vi "最高權限模式test.vi"() -> ()   [LabVIEW 2022 SP3]
panel:
  out "text":string[](array[string])
  out "Tab Control":enum32{"Page 1", "Page 2", "Page 3", "Page 4"}(tab)
  in  "輸入最高權限帳號:":string
  in  "輸入最高權限密碼:":string
  in  "登入":bool
  in  "Stop Button":bool
  in  "創建使用者帳號":bool
  in  "刪除使用者帳號":bool
  in  "登出":bool
  in  "創建密碼":string
  in  "創建帳號":string
  in  "創建建立":bool
  in  "創建離開":bool
  in  "Combo Box":string(combo)
  in  "刪除離開":bool
  in  "確認刪除":bool
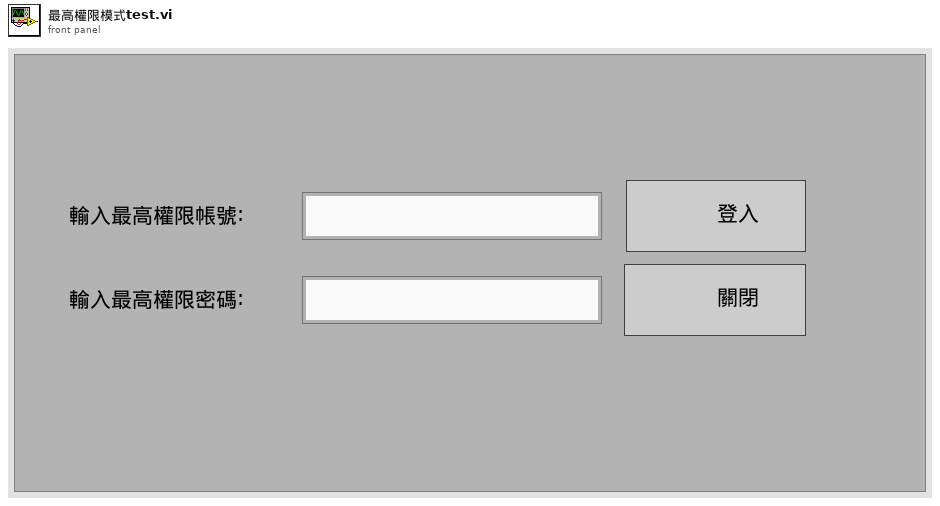
[diagram p1: front panel]
types:
  T1 = typedef "最高權限Control.ctl" = enum16{"刪除帳號", "創建帳號", "登出", "登入完成", "初始", "登入", "創建使用者帳密", "刪除使用者帳密", "離開"}
  T2 = enum16{"open", "replace", "create", "open or create", "replace or create", "replace or create with confirmation"}
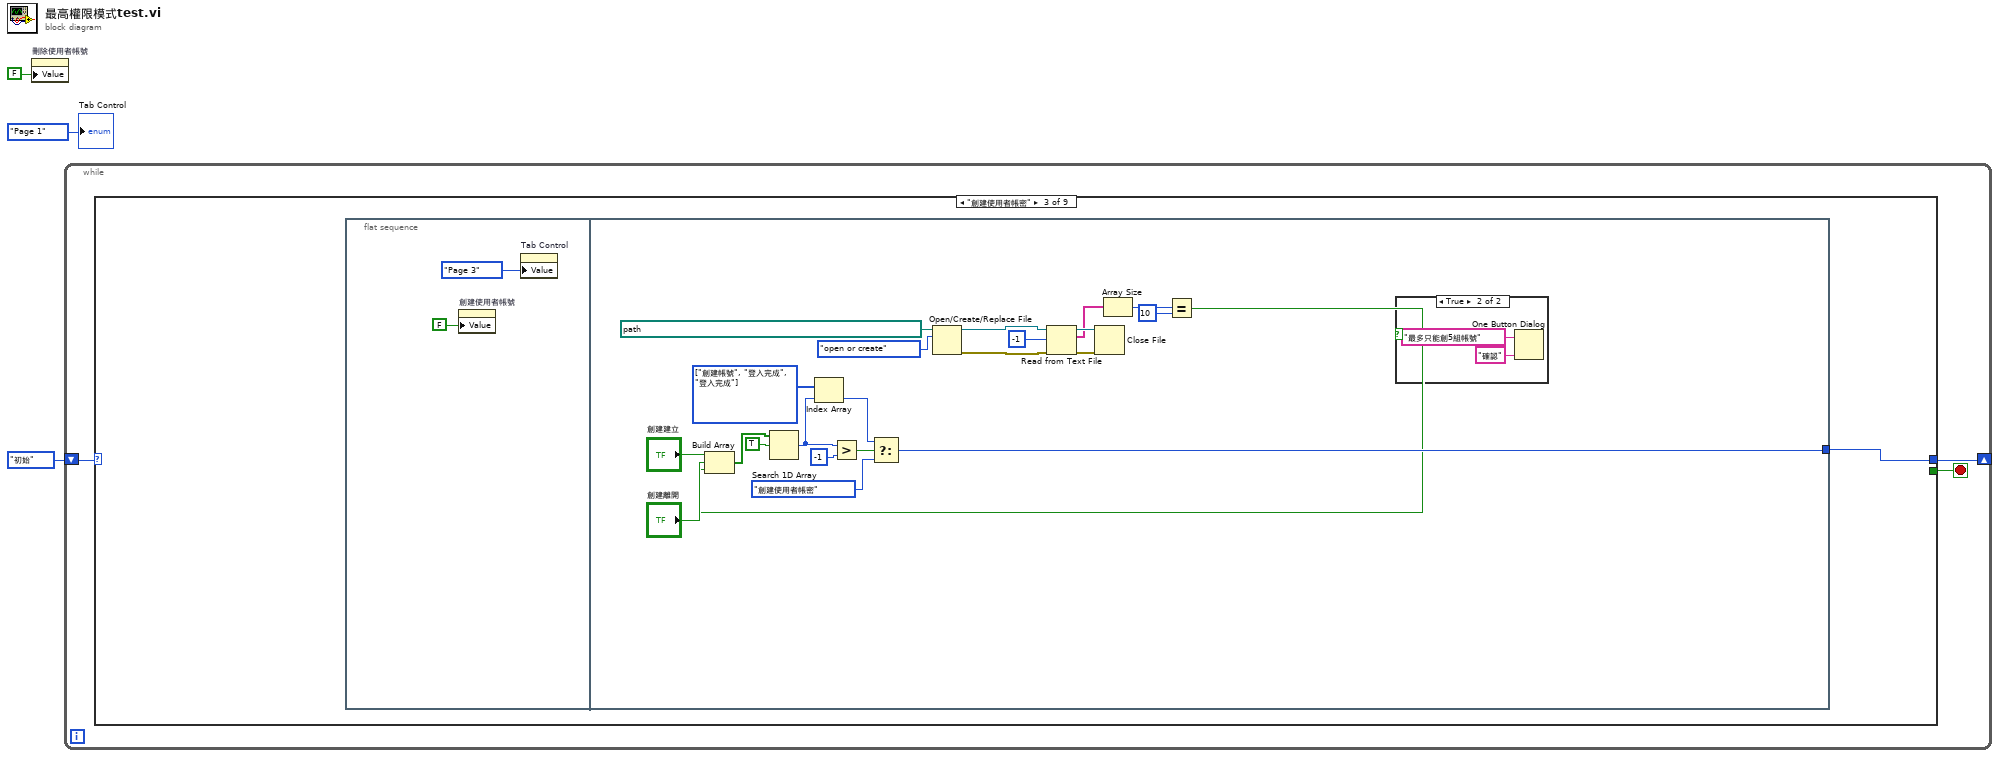
[diagram p0: block diagram]
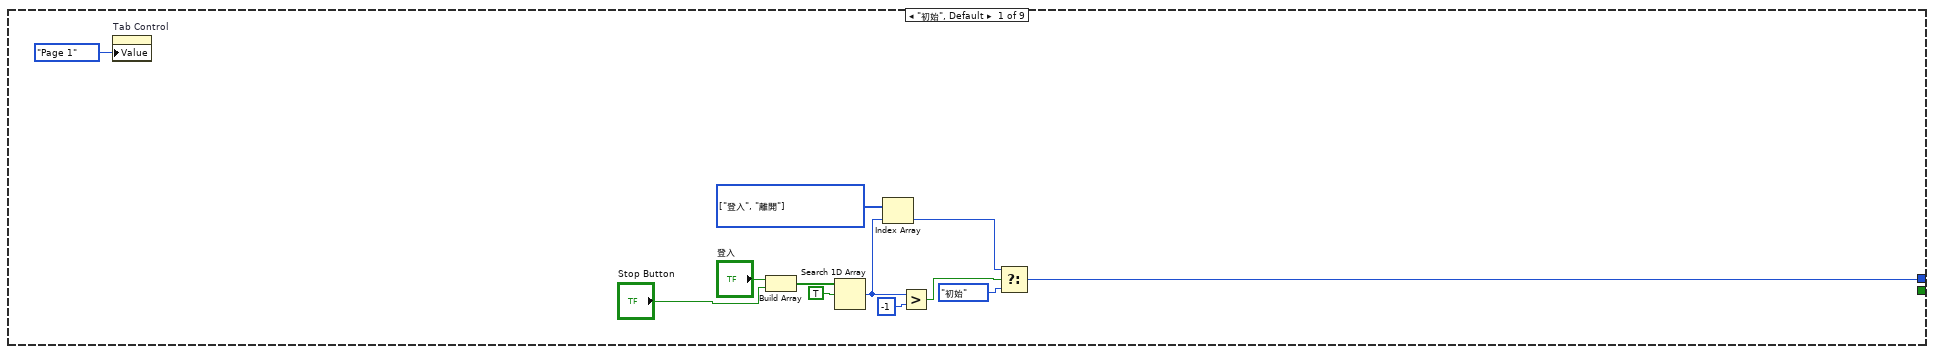
[diagram p2: hidden frame]
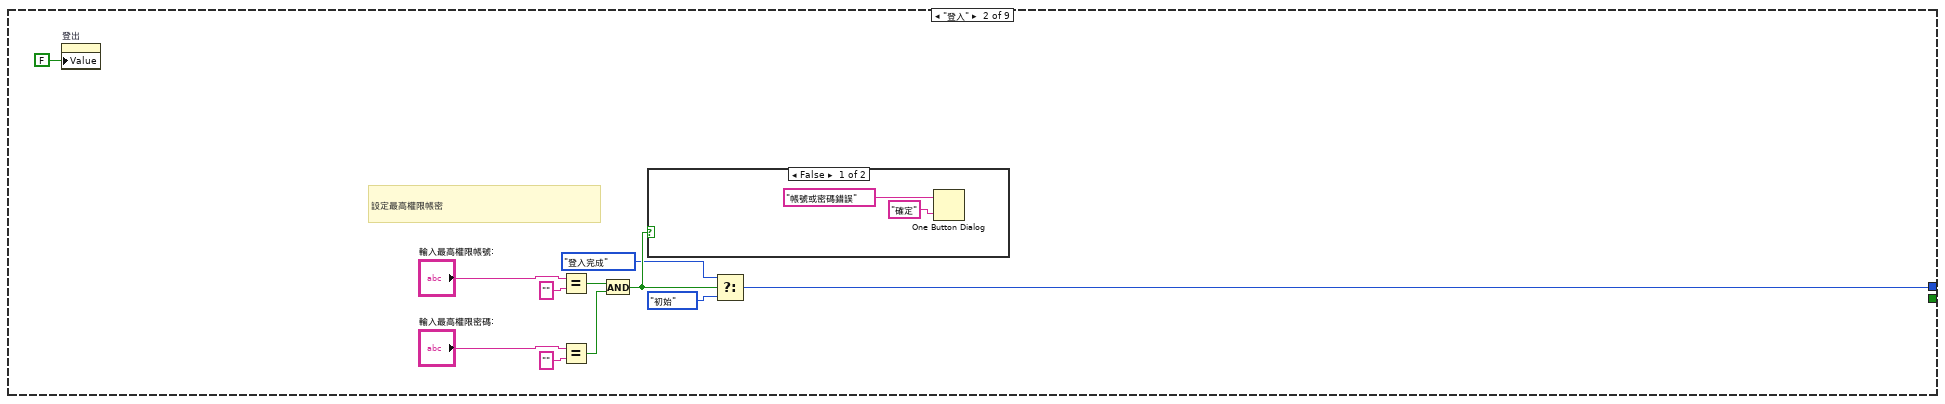
[diagram p3: hidden frame]
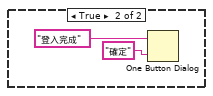
[diagram p4: hidden frame]
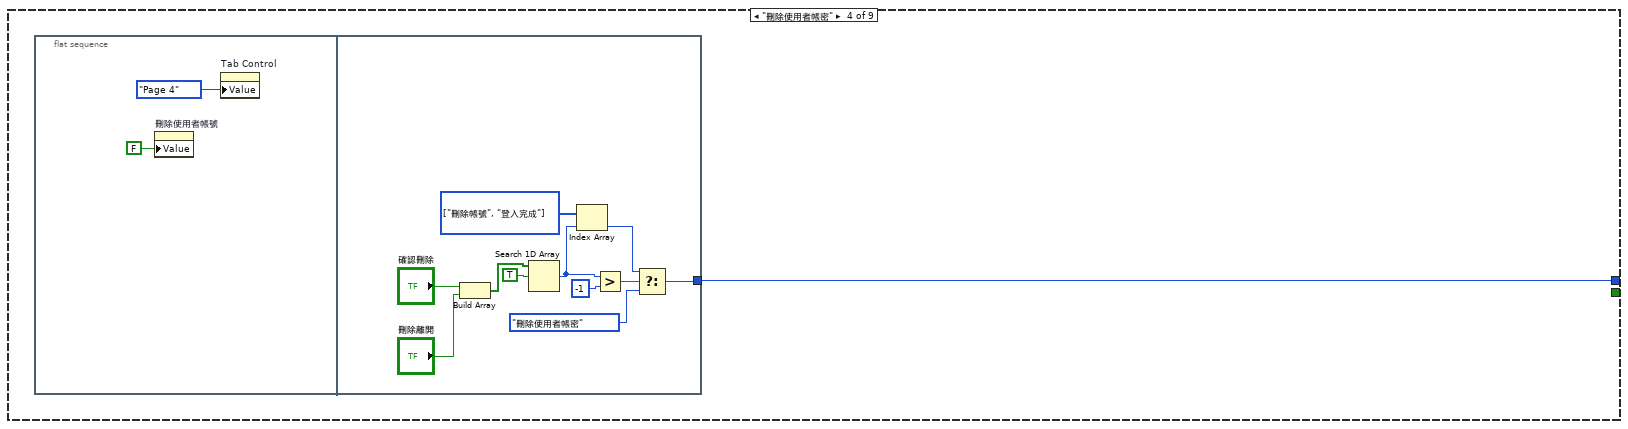
[diagram p6: hidden frame]
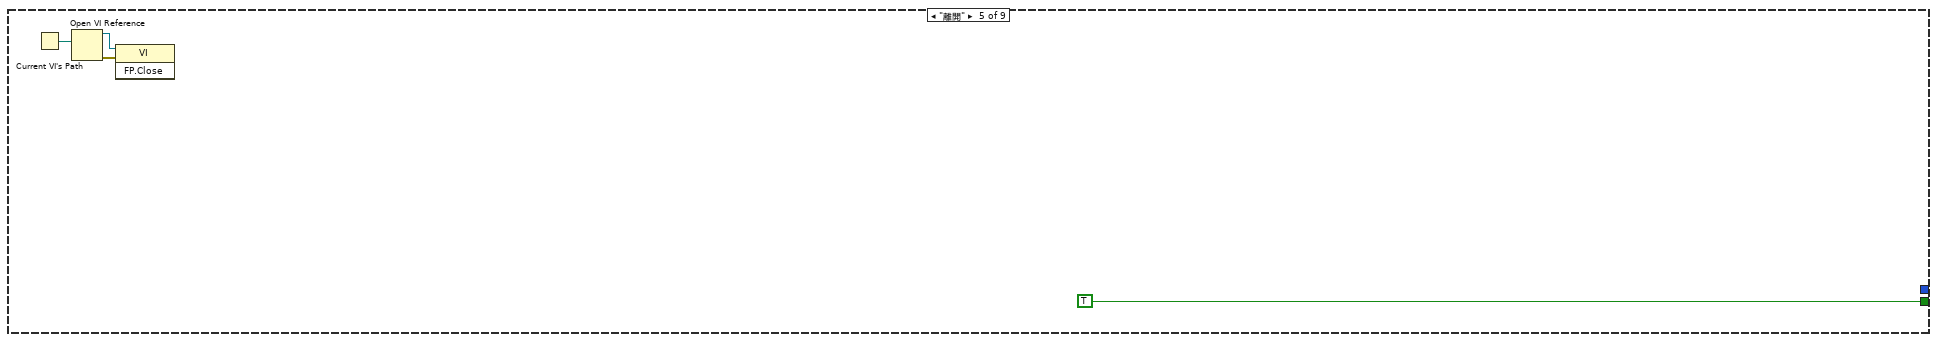
[diagram p7: hidden frame]
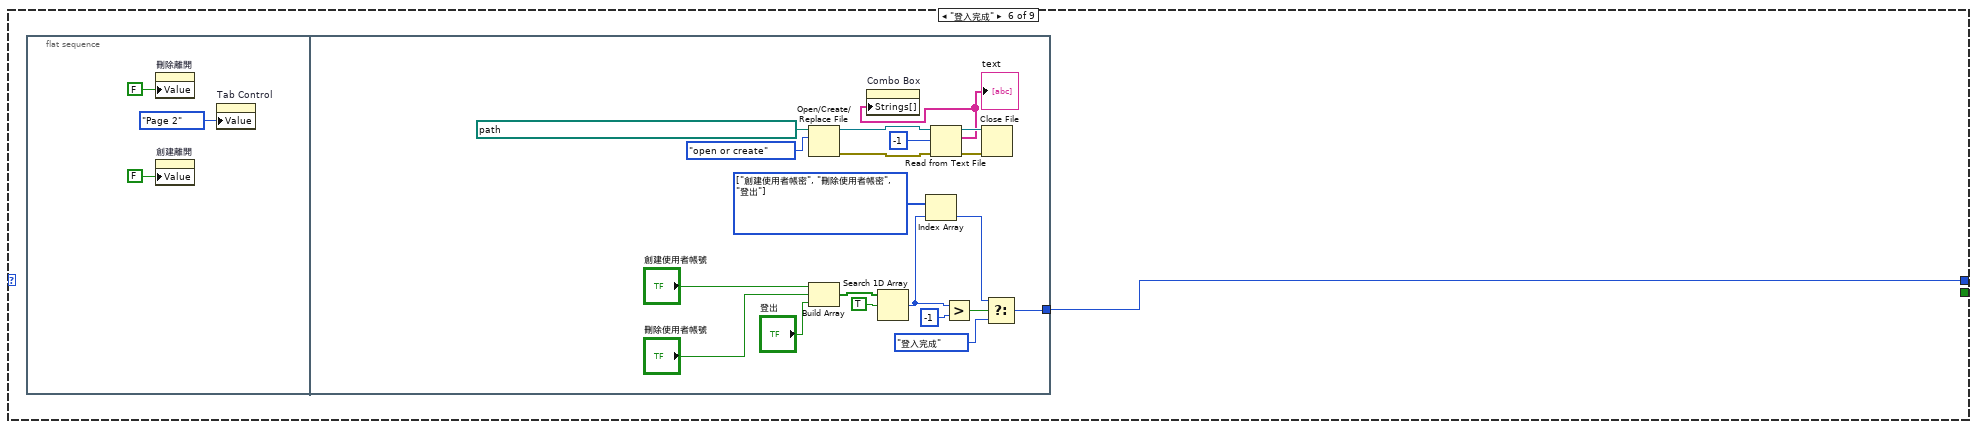
[diagram p8: hidden frame]
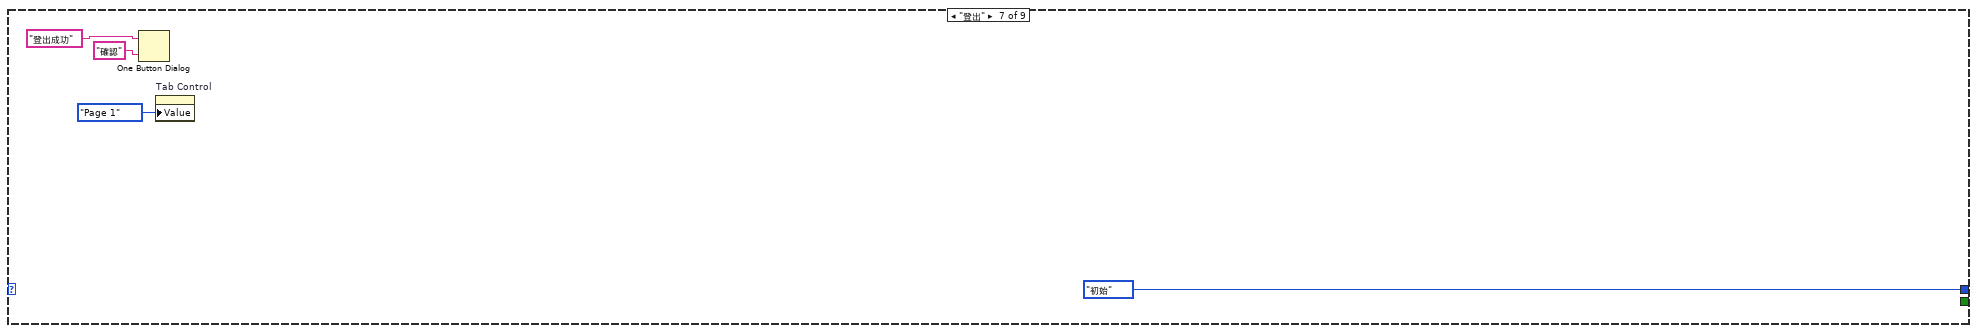
[diagram p9: hidden frame]
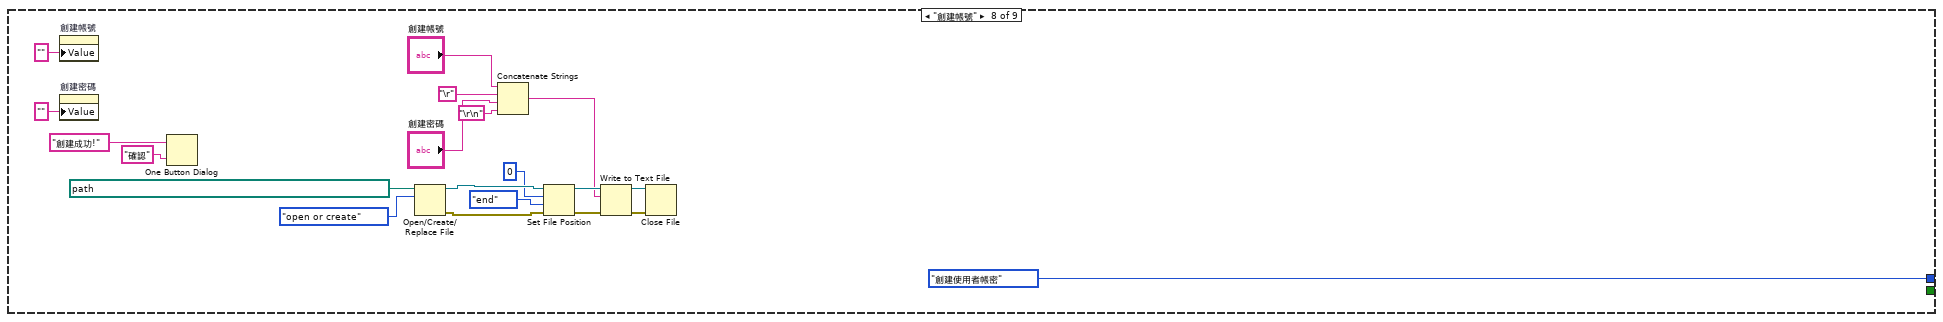
[diagram p10: hidden frame]
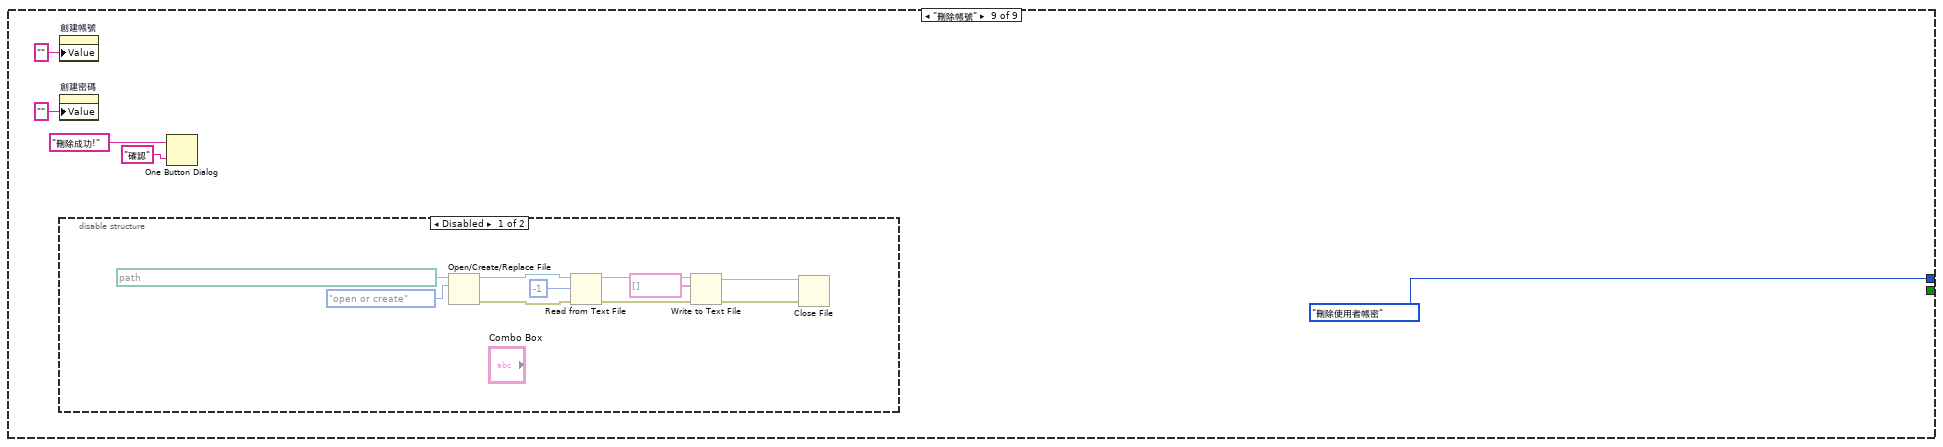
[diagram p11: hidden frame]
diagram:
  n1 = property on="刪除使用者帳號" class="Bool (strict)"("Value"=FALSE ("刪除使用者帳號")) -> ()  [unwired: 2 in, 2 out]
  n2 = while {
    shift-right: [w5] -> _
    shift-left: 最高權限Control."初始" -> [w6]
    stop <- w4 stop-if-true
    n3 = case shown="\"創建使用者帳密\"" w6 {
      tunnel: [w9 w20 w34 w61 _ w79 最高權限Control."初始" 最高權限Control."創建使用者帳密" 最高權限Control."刪除使用者帳密"] -> w5
      tunnel: [_ _ _ _ TRUE _ _ _ _] -> w4
      frame "初始", Default {
        w14 = T1[] [enum."登入", enum."離開"] items=["刪除帳號", "創建帳號", "登出", "登入完成", "初始", "登入", "創建使用者帳密", "刪除使用者帳密", "離開"]
        n4 = property on="Tab Control" class="TabCtl (strict)"("Value"=enum32{"Page 1", "Page 2"}."Page 1" ("Tab Control")) -> ()  [unwired: 2 in, 2 out]
        n5 = Build Array("登入", "Stop Button") -> (w16:bool[])
        n6 = Search 1D Array(1D array=w16, element=TRUE) -> (index of element=w13:i32)  [unwired: 1 in]
        n7 = Index Array(array=w14, index=w13) -> (element=w8:T1)
        n8 = Greater?(x=w13, y=-1) -> (0:w11:bool)
        n9 = Select(t=w8, s=w11, f=最高權限Control."初始") -> (s? t:f=w9:T1)
      }
      frame "登入" {
        # "設定最高權限帳密"
        n10 = property on="登出" class="Bool (strict)"("Value"=FALSE ("登出")) -> ()  [unwired: 2 in, 2 out]
        n11 = Equal?(x="輸入最高權限帳號:", y="") -> (x = y?=w25:bool)
        n12 = Equal?(x="輸入最高權限密碼:", y="") -> (x = y?=w24:bool)
        n13 = And(x=w25, y=w24) -> (x .and. y?=w23:bool)
        n14 = case shown="False" w23 {
          frame False {
            n15 = One Button Dialog(message="帳號或密碼錯誤", button name ("OK")="確定") -> ()  [unwired: 1 out]
          }
          frame True {
            n16 = One Button Dialog(message="登入完成", button name ("OK")="確定") -> ()  [unwired: 1 out]
          }
        }
        n17 = Select(t=最高權限Control."登入完成", s=w23, f=最高權限Control."初始") -> (s? t:f=w20:T1)
      }
      frame "創建使用者帳密" {
        n18 = flat-sequence {
          tunnel: [w48] -> w34
          frame #0 {
            n19 = property on="創建使用者帳號" class="Bool (strict)"("Value"=FALSE ("創建使用者帳號")) -> ()  [unwired: 2 in, 2 out]
            n20 = property on="Tab Control" class="TabCtl (strict)"("Value"=enum32{"Page 1", "Page 2", "Page 3", "Page 4"}."Page 3" ("Tab Control")) -> ()  [unwired: 2 in, 2 out]
          }
          frame #1 {
            w49 = T1[] [enum."創建帳號", enum."登入完成", enum."登入完成"] items=["刪除帳號", "創建帳號", "登出", "登入完成", "初始", "登入", "創建使用者帳密", "刪除使用者帳密", "離開"]
            n21 = Open/Create/Replace File(file path (use dialog)=path "C:/Users/kenny/OneDrive/桌面/機械手臂/使用者帳密.txt", operation (0:open)=T2."open or create") -> (refnum out=w44:refnum<file>, error out=w45:errorcluster)  [unwired: 4 in, 1 out]
            n22 = Read from Text File(file (use dialog)=w44, count=-1, error in=w45) -> (refnum out=w47:refnum<file>, text=w40:string[], error out=w46:errorcluster)  [unwired: 1 in, 1 out]
            n23 = Close File(refnum=w47, error in=w46) -> ()  [unwired: 2 out]
            n24 = Array Size(array=w40) -> (size(s)=w39:i32)
            n25 = Equal?(x=w39, y=10) -> (x = y?=w37:bool)
            n26 = Build Array("創建建立", "創建離開", w37) -> (w58:bool[])
            n27 = Search 1D Array(1D array=w58, element=TRUE) -> (index of element=w57:i32)  [unwired: 1 in]
            n28 = Index Array(array=w49, index=w57) -> (element=w55:T1)
            n29 = Greater?(x=w57, y=-1) -> (0:w56:bool)
            n30 = Select(t=w55, s=w56, f=最高權限Control."創建使用者帳密") -> (s? t:f=w48:T1)
            n31 = case shown="True" w37 {
              frame False {
              }
              frame True {
                n32 = One Button Dialog(message="最多只能創5組帳號", button name ("OK")="確認") -> ()  [unwired: 1 out]
              }
            }
          }
        }
      }
      frame "刪除使用者帳密" {
        n33 = flat-sequence {
          tunnel: [w64] -> w61
          frame #0 {
            n34 = property on="刪除使用者帳號" class="Bool (strict)"("Value"=FALSE ("刪除使用者帳號")) -> ()  [unwired: 2 in, 2 out]
            n35 = property on="Tab Control" class="TabCtl (strict)"("Value"=enum32{"Page 1", "Page 2", "Page 3", "Page 4"}."Page 4" ("Tab Control")) -> ()  [unwired: 2 in, 2 out]
          }
          frame #1 {
            w65 = T1[] [enum."刪除帳號", enum."登入完成"] items=["刪除帳號", "創建帳號", "登出", "登入完成", "初始", "登入", "創建使用者帳密", "刪除使用者帳密", "離開"]
            n36 = Build Array("確認刪除", "刪除離開") -> (w71:bool[])
            n37 = Search 1D Array(1D array=w71, element=TRUE) -> (index of element=w72:i32)  [unwired: 1 in]
            n38 = Index Array(array=w65, index=w72) -> (element=w74:T1)
            n39 = Greater?(x=w72, y=-1) -> (0:w73:bool)
            n40 = Select(t=w74, s=w73, f=最高權限Control."刪除使用者帳密") -> (s? t:f=w64:T1)
          }
        }
      }
      frame "離開" {
        n41 = Current VI's Path() -> (path=w75:path)
        n42 = Open VI Reference(vi path=w75) -> (vi reference=w77:refnum<vi>, error out=w76:errorcluster)  [unwired: 5 in]
        n43 = invoke class="VI" method="FP.Close"(reference=w77, error in=w76) -> ()  [unwired: 1 in, 3 out]
      }
      frame "登入完成" {
        n44 = flat-sequence {
          tunnel: [w91] -> w79
          frame #0 {
            n45 = property on="刪除離開" class="Bool (strict)"("Value"=FALSE ("刪除離開")) -> ()  [unwired: 2 in, 2 out]
            n46 = property on="創建離開" class="Bool (strict)"("Value"=FALSE ("創建離開")) -> ()  [unwired: 2 in, 2 out]
            n47 = property on="Tab Control" class="TabCtl (strict)"("Value"=enum32{"Page 1", "Page 2"}."Page 2" ("Tab Control")) -> ()  [unwired: 2 in, 2 out]
          }
          frame #1 {
            w92 = T1[] [enum."創建使用者帳密", enum."刪除使用者帳密", enum."登出"] items=["刪除帳號", "創建帳號", "登出", "登入完成", "初始", "登入", "創建使用者帳密", "刪除使用者帳密", "離開"]
            n48 = Open/Create/Replace File(file path (use dialog)=path "C:/Users/kenny/OneDrive/桌面/機械手臂/使用者帳密.txt", operation (0:open)=T2."open or create") -> (refnum out=w87:refnum<file>, error out=w88:errorcluster)  [unwired: 4 in, 1 out]
            n49 = Build Array("創建使用者帳號", "刪除使用者帳號", "登出") -> (w99:bool[])
            n50 = Search 1D Array(1D array=w99, element=TRUE) -> (index of element=w100:i32)  [unwired: 1 in]
            n51 = Index Array(array=w92, index=w100) -> (element=w101:T1)
            n52 = Read from Text File(file (use dialog)=w87, count=-1, error in=w88) -> (refnum out=w90:refnum<file>, text=w83:string[], error out=w89:errorcluster)  [unwired: 1 in, 1 out]
            "text" <- w83
            n53 = property on="Combo Box" class="CmbBox"("Strings[]"=w83) -> ()  [unwired: 2 in, 2 out]
            n54 = Greater?(x=w100, y=-1) -> (0:w102:bool)
            n55 = Close File(refnum=w90, error in=w89) -> ()  [unwired: 2 out]
            n56 = Select(t=w101, s=w102, f=最高權限Control."登入完成") -> (s? t:f=w91:T1)
          }
        }
      }
      frame "登出" {
        n57 = One Button Dialog(message="登出成功", button name ("OK")="確認") -> ()  [unwired: 1 out]
        n58 = property on="Tab Control" class="TabCtl (strict)"("Value"=enum32{"Page 1", "Page 2"}."Page 1" ("Tab Control")) -> ()  [unwired: 2 in, 2 out]
      }
      frame "創建帳號" {
        n59 = property on="創建帳號" class="Str"("Value"="" ("創建帳號")) -> ()  [unwired: 2 in, 2 out]
        n60 = property on="創建密碼" class="Str"("Value"="" ("創建密碼")) -> ()  [unwired: 2 in, 2 out]
        n61 = One Button Dialog(message="創建成功!", button name ("OK")="確認") -> ()  [unwired: 1 out]
        n62 = Open/Create/Replace File(file path (use dialog)=path "C:/Users/kenny/OneDrive/桌面/機械手臂/使用者帳密.txt", operation (0:open)=T2."open or create") -> (refnum out=w118:refnum<file>, error out=w116:errorcluster)  [unwired: 4 in, 1 out]
        n63 = Concatenate Strings("創建帳號", "\r", "創建密碼", "\r\n") -> (w109:string)
        n64 = Set File Position(offset (in bytes) (0)=i64 0, refnum=w118, from (0:start)=enum16{"start", "end", "current"}."end", error in=w116) -> (refnum out=w117:refnum<file>, error out=w115:errorcluster)
        n65 = Write to Text File(file (use dialog)=w117, text=w109, error in=w115) -> (refnum out=w122:refnum<file>, error out=w123:errorcluster)  [unwired: 1 in, 1 out]
        n66 = Close File(refnum=w122, error in=w123) -> ()  [unwired: 2 out]
      }
      frame "刪除帳號" {
        n67 = property on="創建帳號" class="Str"("Value"="" ("創建帳號")) -> ()  [unwired: 2 in, 2 out]
        n68 = property on="創建密碼" class="Str"("Value"="" ("創建密碼")) -> ()  [unwired: 2 in, 2 out]
        n69 = disable-structure shown="Disabled" {
          frame Disabled {
            n70 = Open/Create/Replace File(file path (use dialog)=path "C:/Users/kenny/OneDrive/桌面/機械手臂/使用者帳密.txt", operation (0:open)=T2."open or create") -> (refnum out=w140:refnum<file>, error out=w141:errorcluster)  [unwired: 4 in, 1 out]
            n71 = Read from Text File(file (use dialog)=w140, count=-1, error in=w141) -> (refnum out=w136:refnum<file>, error out=w135:errorcluster)  [unwired: 1 in, 2 out]
            n72 = Write to Text File(file (use dialog)=w136, text=string[] [], error in=w135) -> (refnum out=w133:refnum<file>, error out=w134:errorcluster)  [unwired: 1 in, 1 out]
            n73 = Close File(refnum=w133, error in=w134) -> ()  [unwired: 2 out]
          }
          frame Enabled {
          }
        }
        n74 = One Button Dialog(message="刪除成功!", button name ("OK")="確認") -> ()  [unwired: 1 out]
      }
    }
  }
  "Tab Control" <- enum32{"Page 1", "Page 2"}."Page 1" ("Tab Control")
